vi "Create All Message Queues.vi"(8 "error in (no error)":errorcluster) -> (0 "error out":errorcluster, 3 "Message Queues out":T1)   [LabVIEW 2023, in "Message Queue.lvlib"]
doc: "This VI creates and initializes all the message queues for your application. If your application requires more than one message queue, right-click the \"Message Queues\" constant above and select Open Type Def. Add the new Message Queue(s) to the type definition, then initialize them in this VI."
uses:
  Message Queue.lvlib
  All Message Queues.ctl
  Message Cluster.ctl
  Enqueue Message (Single).vi
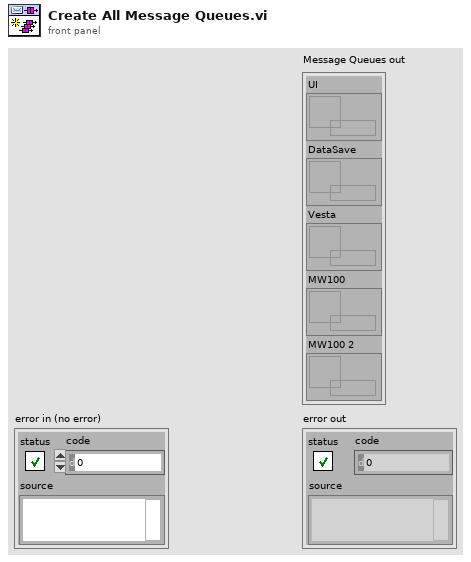
[diagram p1: front panel]
types:
  T1 = typedef "Message Queue.lvlib/All Message Queues.ctl" = cluster{"UI":refnum<queue>, "DataSave":refnum<queue>, "Vesta":refnum<queue>, "MW100":refnum<queue>, "MW100 2":refnum<queue>}
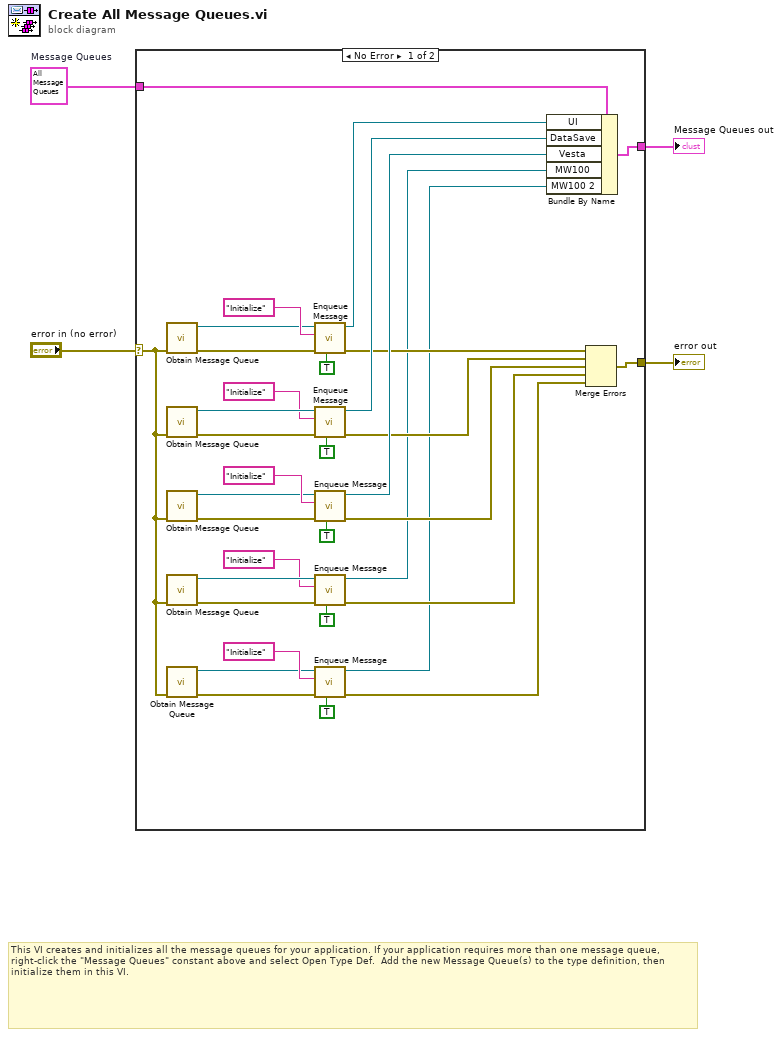
[diagram p0: block diagram]
diagram:
  w2 = T1 {"UI"=refnum, "DataSave"=refnum, "Vesta"=refnum, "MW100"=refnum, "MW100 2"=refnum}  # Message Queues
  # "This VI creates and initializes all the message queues for your application. If your application requires more than one message queue, right-click the \"Message Queues\" constant above and select Open Type Def.  Add the new Message Queue(s) to the type definition, then initialize them in this VI."
  n1 = case shown="No Error" "error in (no error)" {
    selector: "error in (no error)" -> [w7 w40]
    tunnel: [w38 w39] -> w4
    tunnel: w2 -> [w18 w39]
    tunnel: [w19 w40] -> w1
    frame No Error {
      n2 = call "Obtain Message Queue.vi"("error in (no error)"=w7) -> ("error out"=w37:errorcluster, "Message Queue"=w35:refnum<queue>)  [unwired: 9 in]
      n3 = call "Obtain Message Queue.vi"("error in (no error)"=w7) -> ("error out"=w29:errorcluster, "Message Queue"=w31:refnum<queue>)  [unwired: 9 in]
      n4 = call "Obtain Message Queue.vi"("error in (no error)"=w7) -> ("error out"=w28:errorcluster, "Message Queue"=w26:refnum<queue>)  [unwired: 9 in]
      n5 = call "Obtain Message Queue.vi"("error in (no error)"=w7) -> ("error out"=w14:errorcluster, "Message Queue"=w16:refnum<queue>)  [unwired: 9 in]
      n6 = call "Obtain Message Queue.vi"("error in (no error)"=w7) -> ("error out"=w11:errorcluster, "Message Queue"=w9:refnum<queue>)  [unwired: 9 in]
      n7 = call-poly "Enqueue Message.vi"("Priority Message? (F)"=TRUE, "error in (no error)"=w37, "Message"="Initialize", "Message Queue"=w35) -> ("error out"=w22:errorcluster, "dup Message Queue"=w33:refnum<queue>)  [unwired: 6 in]
      n8 = call-poly "Enqueue Message.vi"("Priority Message? (F)"=TRUE, "error in (no error)"=w29, "Message"="Initialize", "Message Queue"=w31) -> ("error out"=w21:errorcluster, "dup Message Queue"=w24:refnum<queue>)  [unwired: 6 in]
      n9 = call-poly "Enqueue Message.vi"("Priority Message? (F)"=TRUE, "error in (no error)"=w28, "Message"="Initialize", "Message Queue"=w26) -> ("error out"=w20:errorcluster, "dup Message Queue"=w23:refnum<queue>)  [unwired: 6 in]
      n10 = call-poly "Enqueue Message.vi"("Priority Message? (F)"=TRUE, "error in (no error)"=w14, "Message"="Initialize", "Message Queue"=w16) -> ("error out"=w12:errorcluster, "dup Message Queue"=w13:refnum<queue>)  [unwired: 6 in]
      n11 = call-poly "Enqueue Message.vi"("Priority Message? (F)"=TRUE, "error in (no error)"=w11, "Message"="Initialize", "Message Queue"=w9) -> ("error out"=w5:errorcluster, "dup Message Queue"=w6:refnum<queue>)  [unwired: 6 in]
      n12 = Bundle By Name(cluster=w18, "UI"=w33, "DataSave"=w24, "Vesta"=w23, "MW100"=w13, "MW100 2"=w6) -> (w38:T1)
      n13 = Merge Errors(w22, w21, w20, w12, w5) -> (w19:errorcluster)
    }
    frame Error {
    }
  }
  "Message Queues out" <- w4
  "error out" <- w1
